vi "Read SV Data.vi"(8 "error in (no error)":errorcluster, 11 "PAS Control in":refnum<class "PAS Control.lvclass">) -> (0 "error out":errorcluster, 2 "SV Data":refnum<k21>="ni.var.psp://rt pxi target/PAS_Var/Data", 3 "PAS Control out":refnum<class "PAS Control.lvclass">)   [LabVIEW 2012, in "PAS Control.lvclass"]
uses:
  PAS Control.lvclass
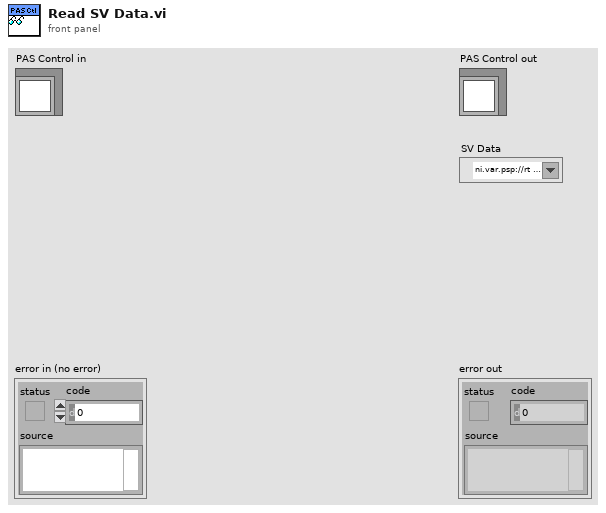
[diagram p1: front panel]
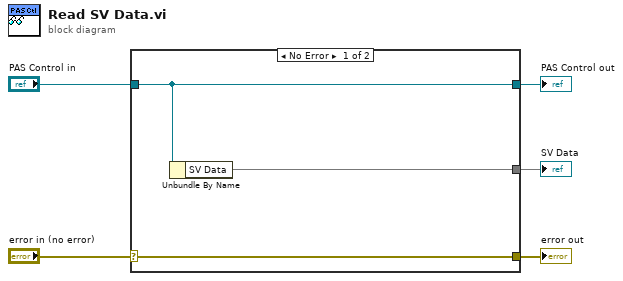
[diagram p0: block diagram]
diagram:
  n1 = case shown="No Error" "error in (no error)" {
    selector: "error in (no error)" -> [w8 w9]
    tunnel: [w8 w9] -> w4
    tunnel: [w7 w10] -> w2
    tunnel: "PAS Control in" -> [w7 w10]
    tunnel: [w6 _] -> w1
    frame No Error {
      n2 = Unbundle By Name(w7) -> ("SV Data"=w6)
    }
    frame Error {
    }
  }
  "error out" <- w4
  "PAS Control out" <- w2
  "SV Data" <- w1
